vi "Get Value String Array from HashTable.vi"(8 "error in (no error)":errorcluster caption="错误输入（无错误）", 10 "Name":string[](array[string]), 11 "Contstant Base 输入":refnum<class "Tag Data.lvclass"> caption="DNL_LabVIEW Object in") -> (0 "error out":errorcluster caption="错误输出", 2 "Value":string[](array[string]), 3 "Contstant Base 输出":refnum<class "Tag Data.lvclass"> caption="DNL_LabVIEW Object out")   [LabVIEW 2013, in "Tag Data.lvclass"]
uses:
  Tag Data.lvclass
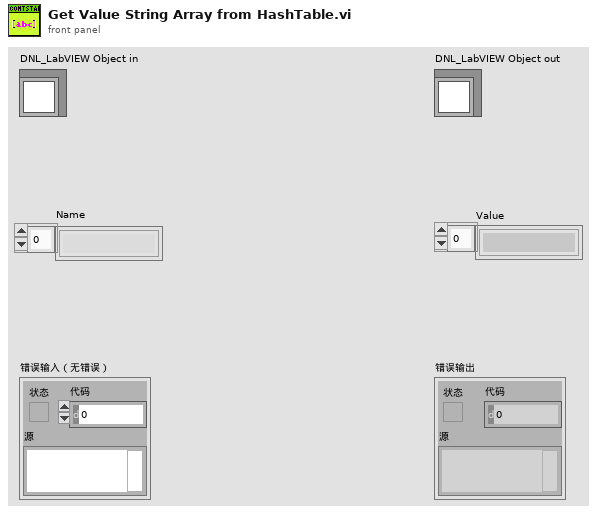
[diagram p1: front panel]
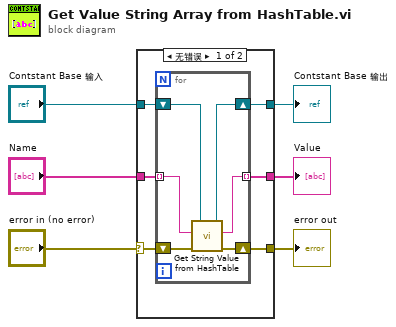
[diagram p0: block diagram]
diagram:
  n1 = case shown="无错误" "error in (no error)" {
    selector: "error in (no error)" -> [w9 w20]
    tunnel: [w8 w20] -> w5
    tunnel: [w11 w19] -> w3
    tunnel: "Contstant Base 输入" -> [w12 w19]
    tunnel: "Name" -> [w10 _]
    tunnel: [w7 _] -> w1
    frame No Error {
      n2 = for {
        shift-right: [w17] -> w11
        shift-left: w12 -> [w18]
        tunnel: w10 -> [w16] mode=indexing
        tunnel: [w13] -> w7 mode=indexing
        shift-right: [w14] -> w8
        shift-left: w9 -> [w15]
        n3 = call "Get String Value from HashTable.vi"("error in (no error)"=w15, "Name"=w16, "Contstant Base 输入"=w18) -> ("error out"=w14:errorcluster, "Value"=w13:string, "Contstant Base 输出"=w17:refnum<class "Tag Data.lvclass">)  [unwired: 6 in]
      }
    }
    frame Error {
    }
  }
  "error out" <- w5
  "Contstant Base 输出" <- w3
  "Value" <- w1
